vi "Golander pump 2 flows(mL per s, mL per rev) old.vi"(4 "State":i16, 5 "Time":dbl format="%.2f", 6 "Sensor Values":dbl[](array[numeric]), 7 "Set Points":dbl[](array[numeric])=[12.0, 1.0, 1.0, 1.0]) -> (0 "required data":T4={"Set Point names"=["com port", "pump address", "on state 1 (167= states 1, 6, 7)", "on state 2 (23= states 2, 3)", "pump (mL/rev)", "flow 1 (mL/s)", "flow 2 (mL/s)"], "required number of setpoints"=7, "required number of sensors"=0, "Sensor names"=[]}, 3 "output value":dbl)   [LabVIEW 2019]
uses:
  pump 2 flows.ctl
  Pump updates.ctl
  modbusrtu/MB Serial Master Query Write Multiple Registers (poly).vi
panel:
  out "Pump cmd array":T1[](array[typedef])
  out "Pump updates":T2[](array[typedef]) {"Update Time" format="%.2f"}
  in  "Pump updates":T2 {"Update Time" format="%.2f"}
  in  "Timeout":u32=240
  in  "write interval (s)":dbl=5.0
  out "output cluster":T3
  in  "Pump cmds":T1
  in  "error in (no error)":errorcluster
  out "VISA out":refnum<visa-resource-name>
  out "error out":errorcluster
  # "failure at 80 ms"
  # "Enter the correct information for this control code in the required data structure below. Then make the current value default by right clicking on the border of the data structure. Select \"data operations\" and then select \"make current value default\". These values will be displayed by process controller."
  # "Mode: RTU\nAddresses: 1-247 (User Defined)\nBaud Rate: 9600\nData Bits: 8\nCRC: Even Parity\nStop Bit: 1"
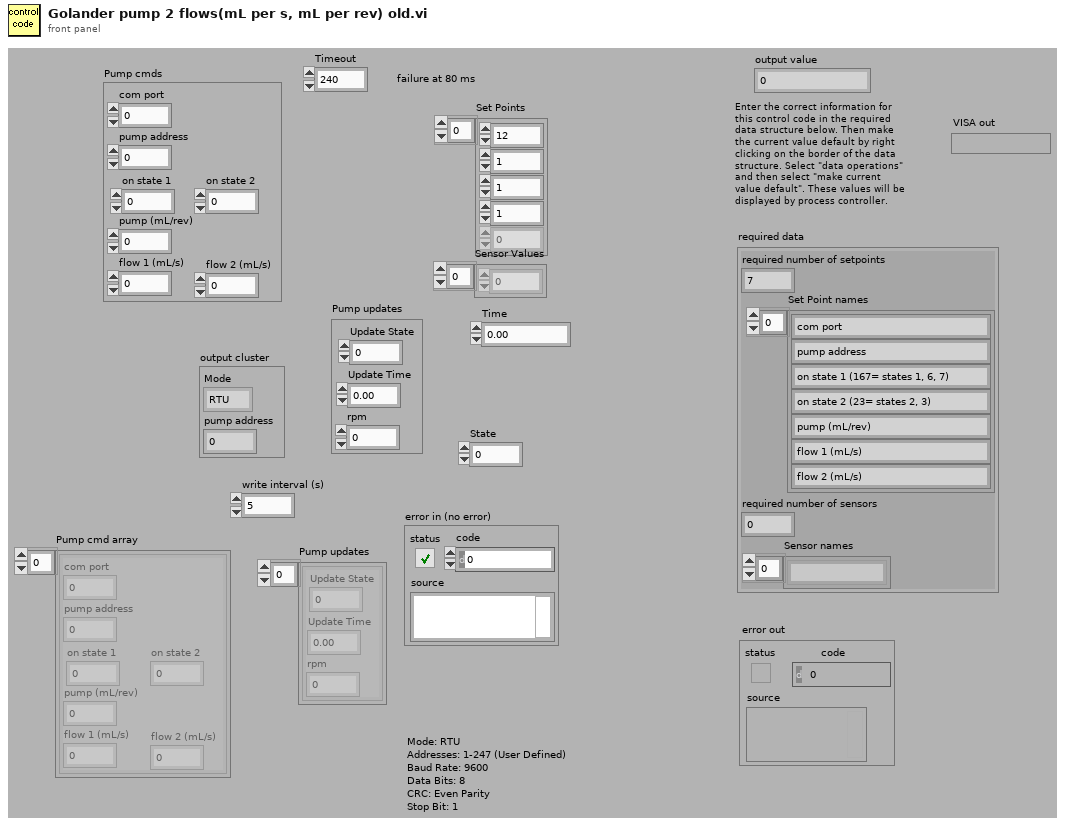
[diagram p1: front panel]
types:
  T1 = typedef "pump 2 flows.ctl" = cluster{"com port":u8, "pump address":u8, "on state 1":i32, "on state 2":i32, "pump (mL/rev)":dbl, "flow 1 (mL/s)":dbl, "flow 2 (mL/s)":dbl}
  T2 = typedef "Pump updates.ctl" = cluster{"Update State":i16, "Update Time":dbl, "rpm":dbl}
  T3 = cluster{"Mode":enum16{"RTU", "ASCII"}, "pump address":u8}
  T4 = cluster{"Set Point names":string[], "required number of setpoints":u8, "required number of sensors":u8, "Sensor names":string[]}
  T5 = cluster{"Set Points[0]":dbl, "Set Points[1]":dbl, "Set Points[2]":dbl, "Set Points[3]":dbl, "Set Points[4]":dbl, "Set Points[5]":dbl, "Set Points[6]":dbl}
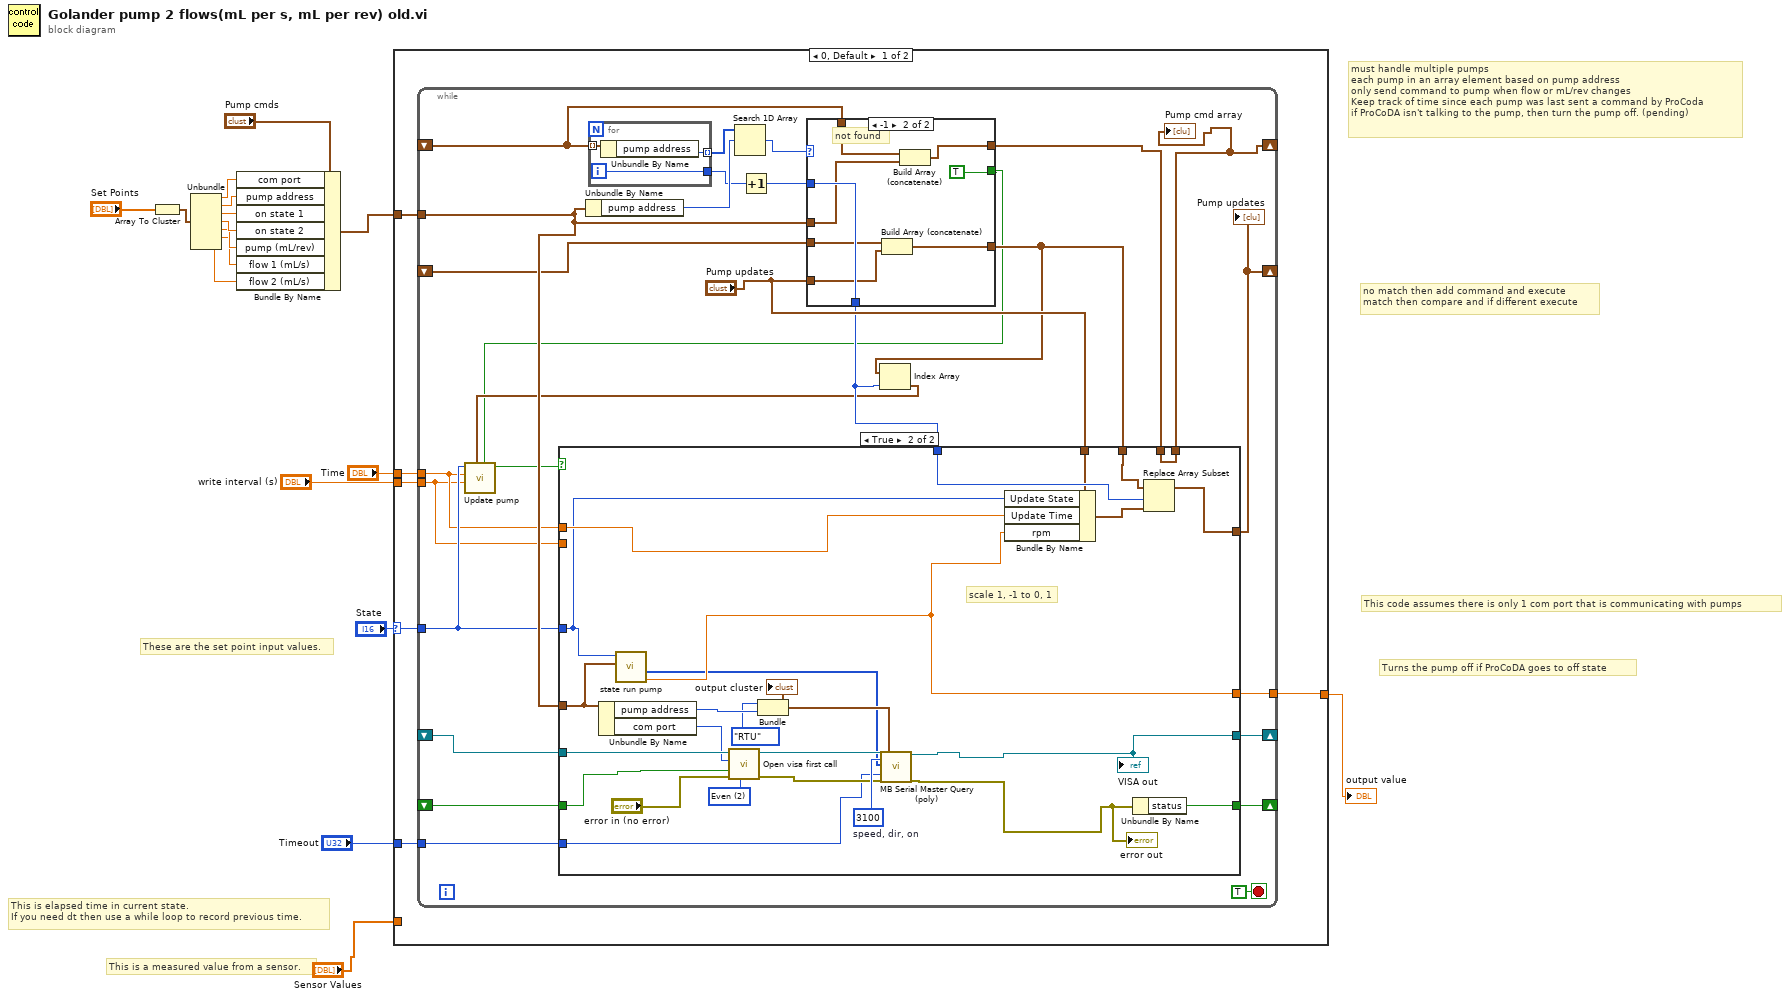
[diagram p0: block diagram]
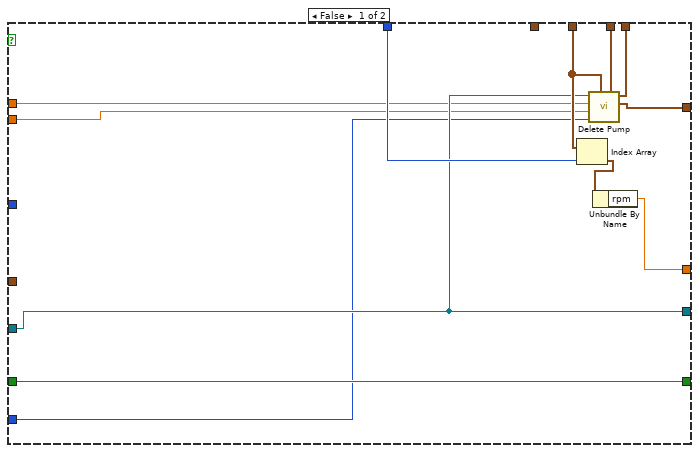
[diagram p2: hidden frame]
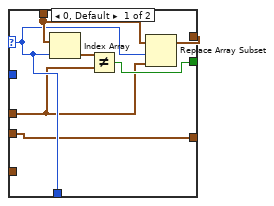
[diagram p3: hidden frame]
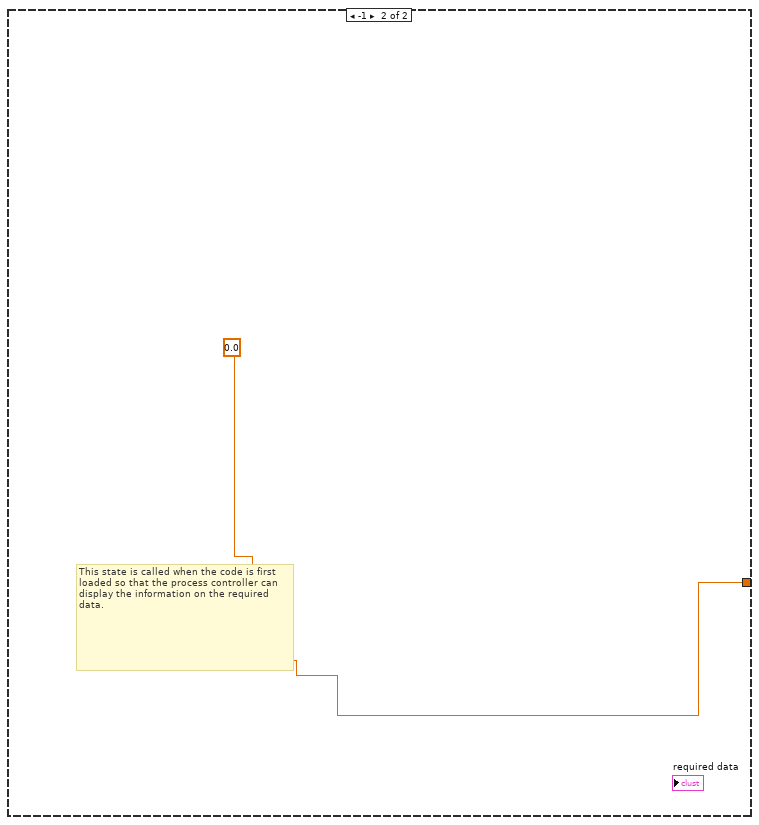
[diagram p4: hidden frame]
diagram:
  # "Turns the pump off if ProCoDA goes to off state"
  # "This code assumes there is only 1 com port that is communicating with pumps"
  # "no match then add command and execute\nmatch then compare and if different execute"
  # "must handle multiple pumps\neach pump in an array element based on pump address\nonly send command to pump when flow or mL/rev changes\nKeep track of time since each pump was last sent a command by ProCoda\nif ProCoDA isn't talking to the pump, then turn the pump off. (pending)"
  # "These are the set point input values."
  # "This is a measured value from a sensor."
  # "This is elapsed time in current state.\nIf you need dt then use a while loop to record previous time."
  n1 = Array To Cluster(array="Set Points") -> (cluster=w14:T5)
  n2 = Unbundle(w14) -> ("Set Points[0]"=w10:dbl, "Set Points[1]"=w15:dbl, "Set Points[2]"=w7:dbl, "Set Points[3]"=w4:dbl, "Set Points[4]"=w3:dbl, "Set Points[5]"=w2:dbl, "Set Points[6]"=w1:dbl)
  n3 = Bundle By Name(cluster="Pump cmds", "com port"=w10, "pump address"=w15, "on state 1"=w7, "on state 2"=w4, "pump (mL/rev)"=w3, "flow 1 (mL/s)"=w2, "flow 2 (mL/s)"=w1) -> (w12:T1)
  n4 = case shown="0, Default" "State" {
    selector: "State" -> [w21 _]
    tunnel: [w22 0.0 ("fraction on")] -> w9
    tunnel: w12 -> [w23 _]
    tunnel: "Sensor Values" -> [_ _]
    tunnel: "Time" -> [w20 _]
    tunnel: "write interval (s)" -> [w19 _]
    tunnel: "Timeout" -> [w18 _]
    frame 0, Default {
      n5 = while {
        shift-right: [w46] -> _
        shift-left: _ -> [w49]
        tunnel: w23 -> [w38]
        shift-right: [w47] -> _
        shift-left: _ -> [w48]
        shift-right: [w24] -> _
        shift-left: _ -> [w41]
        tunnel: w21 -> [w32]
        tunnel: w20 -> [w31]
        shift-right: [w36] -> _
        shift-left: _ -> [w37]
        tunnel: w19 -> [w25]
        tunnel: [w45] -> w22
        tunnel: w18 -> [w27]
        stop <- TRUE stop-if-true
        n6 = Unbundle By Name(w38) -> ("pump address"=w43:u8)
        n7 = for {
          tunnel: [w106] -> w44 mode=indexing
          tunnel: w41 -> [w105] mode=indexing
          tunnel: [w104] -> w40
          i -> [w104]
          n8 = Unbundle By Name(w105) -> ("pump address"=w106:u8)
        }
        n9 = Search 1D Array(1D array=w44, element=w43) -> (index of element=w42:i32)  [unwired: 1 in]
        n10 = Increment(x=w40) -> (x+1=w39:i32)
        n11 = case shown="-1" w42 {
          selector: w42 -> [w91 _]
          tunnel: [w94 TRUE] -> w28
          tunnel: w41 -> [w93 w102]
          tunnel: [w92 w101] -> w26
          tunnel: w39 -> [_ w100]
          tunnel: [w91 w100] -> w34
          tunnel: w38 -> [w90 w99]
          tunnel: w37 -> [w89 w98]
          tunnel: [w89 w97] -> w33
          tunnel: "Pump updates" -> [_ w96]
          frame 0, Default {
            n12 = Index Array(array=w93, index=w91) -> (element=w95:T1)
            n13 = Not Equal?(x=w95, y=w90) -> (x != y?=w94:bool)
            n14 = Replace Array Subset(array=w93, new element=w90, index=w91) -> (w92:T1[])
          }
          frame -1 {
            # "not found"
            n15 = Build Array (concatenate)(w98, w96) -> (w97:T2[])
            n16 = Build Array (concatenate)(w102, w99) -> (w101:T1[])
          }
        }
        n17 = Index Array(array=w33, index=w34) -> (element=w30:T2)
        n18 = call "Update pump.vi"("new pump cmd"=w28, "Pump updates"=w30, "write interval (s)"=w25, "Time"=w31, "State"=w32) -> ("update"=w29:bool)  [unwired: 6 in]
        n19 = case shown="True" w29 {
          tunnel: w49 -> [w54 w87]
          tunnel: w48 -> [w62 w65]
          tunnel: [w62 w86] -> w47
          tunnel: [w54 w63] -> w46
          tunnel: [w59 w68] -> w45
          tunnel: w38 -> [_ w75]
          tunnel: w32 -> [_ w67]
          tunnel: w31 -> [w53 w72]
          tunnel: [w57 w76] -> w36
          tunnel: w33 -> [w58 w77]
          tunnel: w34 -> [w61 w73]
          tunnel: "Pump updates" -> [_ w71]
          tunnel: w27 -> [w52 w70]
          tunnel: w26 -> [w56 w69]
          tunnel: [w55 w69] -> w24
          tunnel: w25 -> [w51 _]
          frame False {
            n20 = Index Array(array=w58, index=w61) -> (element=w60:T2)
            n21 = call "Delete Pump.vi"("pump cmd array"=w56, "Pump updates"=w58, "Timeout"=w52, "write interval (s)"=w51, "Time"=w53, "VISA"=w54) -> ("Pump updates out"=w57:T2[], "pump cmd array out"=w55:T1[])  [unwired: 4 in]
            n22 = Unbundle By Name(w60) -> ("rpm"=w59:dbl)
          }
          frame True {
            w78 = u16 2 items=["None", "Odd", "Even", "Mark", "Space"] ("Parity")
            w81 = u16 3100  # speed, dir, on
            # "scale 1, -1 to 0, 1"
            n23 = Unbundle By Name(w75) -> ("pump address"=w83:u8, "com port"=w85:u8)
            n24 = call "state run pump.vi"("pump command"=w75, "State"=w67) -> ("rpm"=w68:dbl, "registers"=w66:u16[])  [unwired: 2 in, 2 out]
            n25 = call "Open visa first call.vi"("Parity"=w78, "error in (no error)"="error in (no error)", "error"=w65, "Com port"=w85, "VISA Refnum in"=w87) -> ("error out"=w80:errorcluster, "VISA Refnum out"=w84:refnum<visa-resource-name>)  [unwired: 5 in]
            n26 = Bundle("Mode"=enum16{"RTU", "ASCII"}."RTU", "pump address"=w83) -> (w79:T3)  [unwired: 1 in]
            "output cluster" <- w79
            n27 = call-poly "MB Serial Master Query (poly).vi"("VISA resource name"=w84, "Starting Address"=w81, "Registers"=w66, "Timeout"=w70, "error in"=w80, "Serial Parameters"=w79) -> ("VISA resource name out"=w63:refnum<visa-resource-name>, "error out"=w64:errorcluster)  [unwired: 11 in, 1 out]
            "VISA out" <- w63
            "error out" <- w64
            n28 = Bundle By Name(cluster=w71, "Update State"=w67, "Update Time"=w72, "rpm"=w68) -> (w74:T2)
            n29 = Unbundle By Name(w64) -> ("status"=w86:bool)
            n30 = Replace Array Subset(array=w77, new element=w74, index=w73) -> (w76:T2[])
          }
        }
        "Pump updates" <- w36
        "Pump cmd array" <- w24
      }
    }
    frame -1 {
      # "This state is called when the code is first loaded so that the process controller can display the information on the required data."
    }
  }
  "output value" <- w9
